vi "UI_VCH.vi"() -> ()   [LabVIEW 2016]
uses:
  <vilib>/Pansino Software/LabVIEW Architecture/Queue Management/PSARC_Queue Valid.vi
  <vilib>/Pansino Software/LabVIEW Architecture/Queue Management/PSARC_Queue Insert Element.vi
  <vilib>/Utility/error.llb/DialogType.ctl
  <vilib>/Pansino Software/LabVIEW Architecture/Queue Management/PSARC_Queue Remove Element.vi
  <vilib>/Pansino Software/LabVIEW Architecture/Queue Management/PSARC_Queue Destroy_Single.vi
  SubVIs/VCH/Private/Ctrls/PSVCH_VCH Status.ctl
  SubVIs/VCH/Private/Ctrls/PSVCH_All Channels.ctl
  SubVIs/VCH/Private/Ctrls/PSVCH_Status.ctl
  <vilib>/Pansino Software/LabVIEW Architecture/Queue Management/PSARC_Queue Create_Single.vi
  DAQ-Config/Controls/PSCHN_Channel Para.ctl
  DAQ-Config/Controls/PSCHN_Card Para.ctl
  <vilib>/Pansino Software/ToolkitLib/Popup Toolkit/Public/PSPOP_Popup Cluster.ctl
panel:
  in  "Caller":string
  in  "View":bool
  in  "Config":bool
  in  "Run":bool
  in  "Pause":bool
  in  "Stop":bool
  in  "Popups":T1 {"Time" format="%<%Y/%m/%d %I:%M:%S>T"; "Boolean" items=["False", "True"]; "Ring" items=["√", "×"]}
  in  "VCH":string(tree)
  out "Message":string caption="信息"
  # "Boolean Colors"
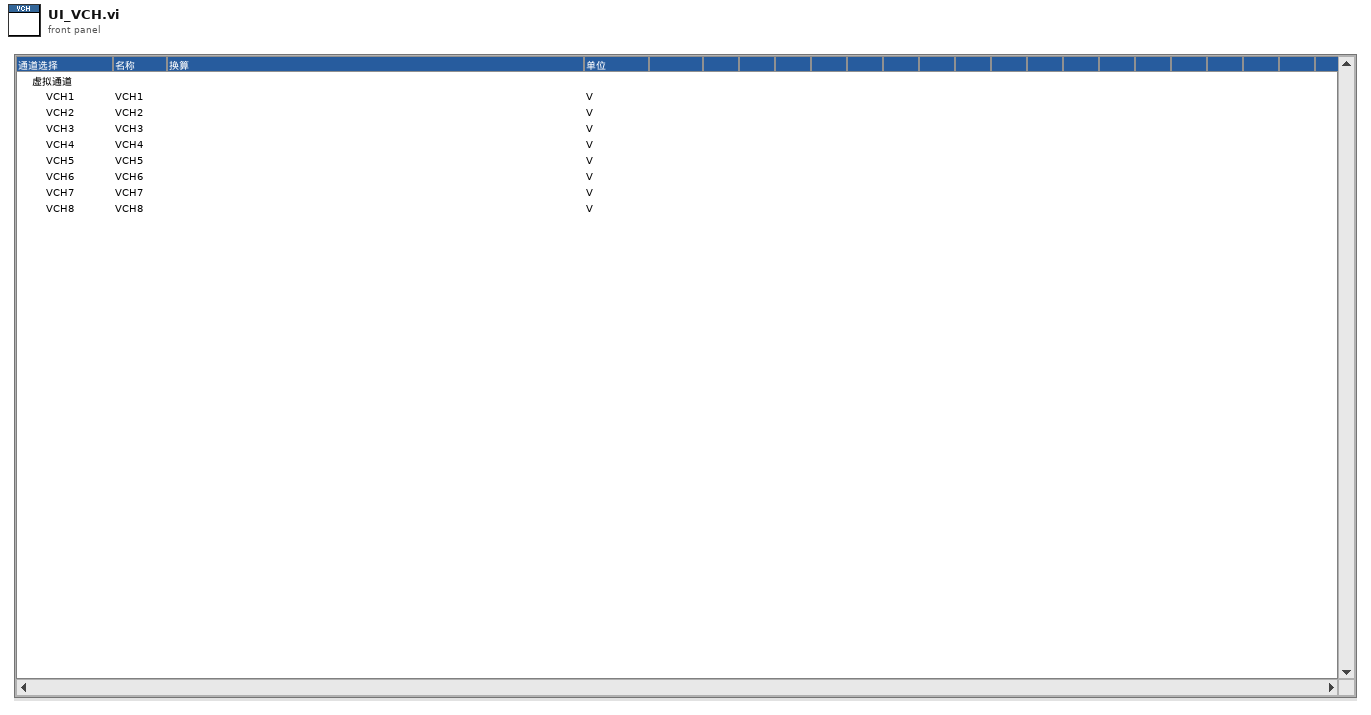
[diagram p1: front panel]
types:
  T1 = typedef "PSPOP_Popup Cluster.ctl" = cluster{"Unknown":bool, "Unknown 2":bool, "String":string, "Integer":i32, "Float":dbl, "Color":u32, "Boolean":u32, "Ring":u32, "Captioned String":cluster{"String":string, "OK":bool, "Cancel":bool}, "Captioned Integer":cluster{"First":i32, "OK":bool, "Cancel":bool}, "Boolean Colors":cluster{"False":cluster{"FG":u32, "BG":u32}, "True":cluster{"FG":u32, "BG":u32}, "T  to  F":cluster{"FG":u32, "BG":u32}, "F  to  T":cluster{"FG":u32, "BG":u32}, "OK":bool, "Cancel":bool}, "2-Int Cluster":cluster{"First":i32, "Second":i32, "OK":bool, "Cancel":bool}, "4-Int Cluster":cluster{"First":i32, "Second":i32, "Third":i32, "Fourth":i32, "OK":bool, "Cancel":bool}, "6-Dbl Cluster":cluster{"First":dbl, "Second":dbl, "Third":dbl, "Fourth":dbl, "Fourth 2":dbl, "Third 2":dbl, "OK":bool, "Cancel":bool}, "Path":path, "Combox":string, "Time":timestamp, "ShortCut":string}
  T2 = typedef "PSVCH_All Channels.ctl" = cluster{"Card Name":string, "Channels Tag":string[], "Channels Name":string[], "Unit":string[]}
  T3 = cluster{"Main Queue":string, "DAQ Queue":string, "ANA Queue":string, "CUI Queue":string, "Q-FocusList":string, "Q-Toolbar":string, "Q-Config":string}
  T4 = cluster{"Error":errorcluster, "Exit":bool, "Local VIRef":refnum<vi>, "Q_Local":cluster{"Name":string, "Order":string, "Data":variant}, "Q_High":cluster{"Name":string, "Order":string, "Data":variant}, "Q_Send":cluster{"Name[]":string[], "Order[]":string[], "Data[]":variant[]}, "Popup Index":i32, "Ref":cluster{"VCHList":refnum<vi>, "Message":refnum<vi>}, "Q_VCHEG":string, "DAQ2ANA":T2[], "PopUp Name":string, "Symbol Path":path}
  T5 = enum8{"Enabled", "Disabled", "Disabled and Grayed Out"}
  T6 = cluster{"Popup Value":variant, "Call Data":variant}
  T7 = typedef "PSVCH_VCH Status.ctl" = cluster{"Tag":string[], "Code[]":i32[], "Dispription[]":string[]}
  T8 = typedef "PSVCH_Status.ctl" = enum16{"Bad", "Stop", "Run", "Pause"}
  T9 = typedef "PSCHN_Card Para.ctl" = cluster{"Module Type":string, "Module Name":string, "ModuSN":string, "ModuIP":string, "Used?":bool, "Connected":bool, "Timing*":cluster{"Sample Rate":dbl}, "Channels":T10[]}
  T10 = typedef "PSCHN_Channel Para.ctl" = cluster{"CHTag*":string, "Used?*":bool, "CHName":string, "Unit":string, "斜率":dbl, "截距":dbl}
  T11 = cluster{"Queue":string, "DAQ Channels":string[]}[]
  T12 = typedef "DialogType.ctl" = u16
  T13 = typedef "PSVCH_VCH Info.ctl" = cluster{"Tag":string[], "Tag String":string[], "Name":string[], "Enable":bool[], "Formula":string[], "Unit":string[], "Save":bool[], "Time":i64[]}
  T14 = cluster{"Tag":string[], "Name":string[], "Type":variant[]}
  T15 = cluster{"VarList":cluster{"Tag":string[], "Name":string[], "Type":variant[]}, "VCH Out":T13}
  T16 = typedef "LVPoint32TypeDef.ctl" = cluster{"Horizontal":i32, "Vertical":i32}
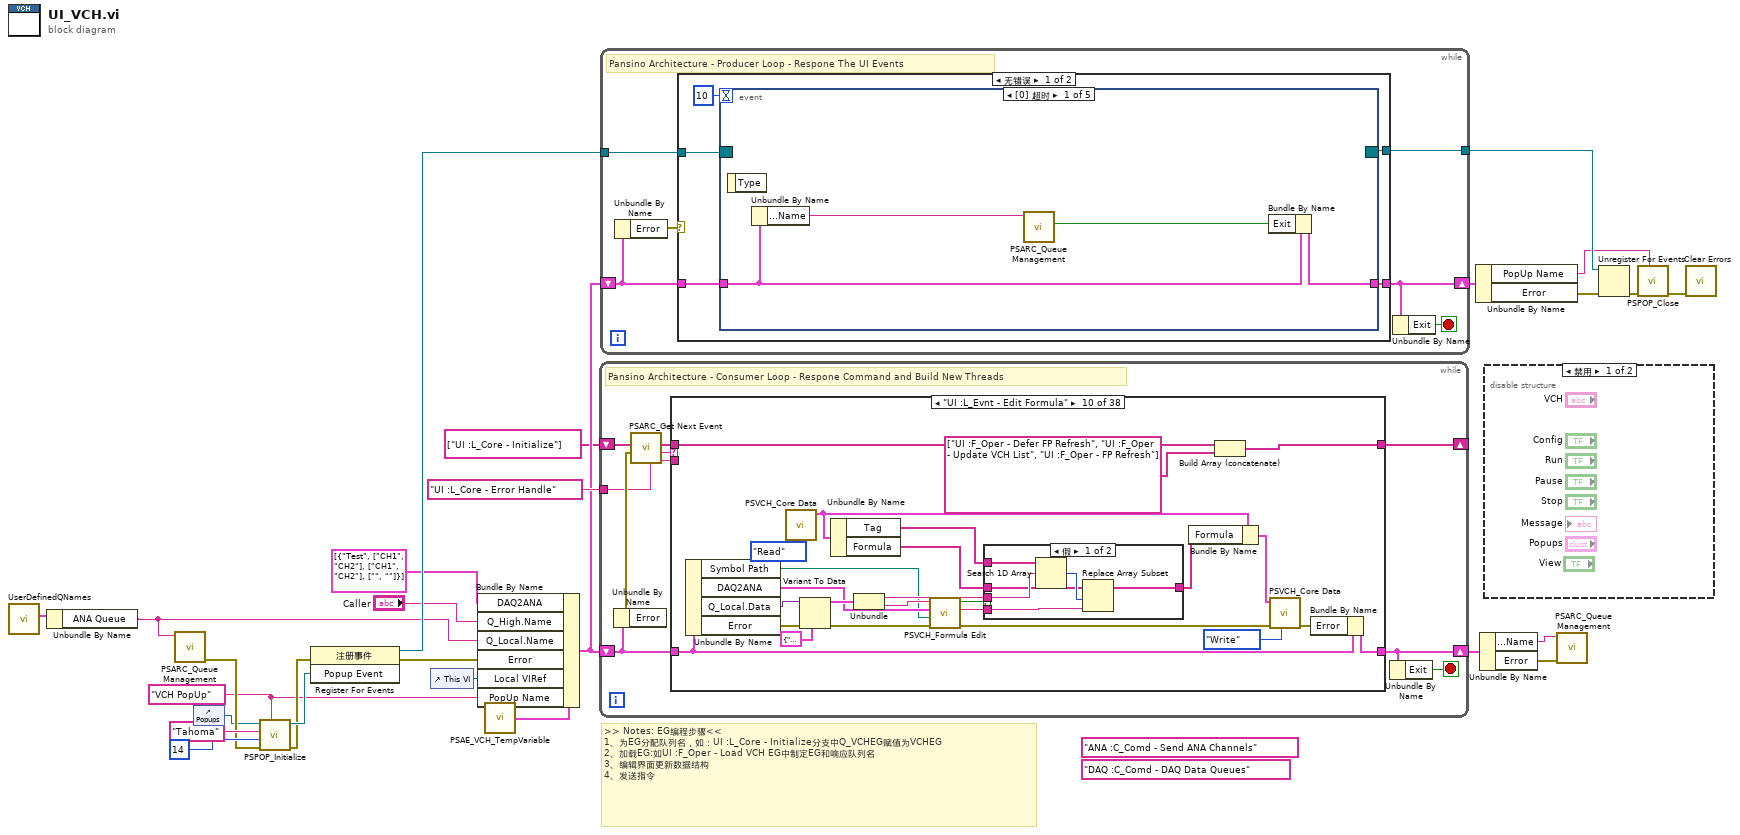
[diagram p0: block diagram]
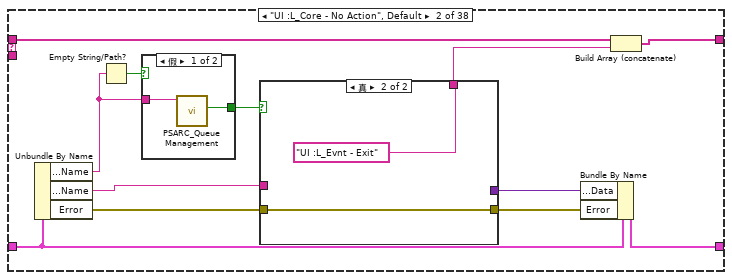
[diagram p4: hidden frame]
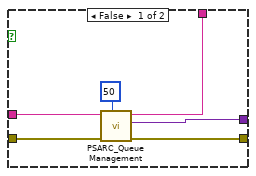
[diagram p6: hidden frame]
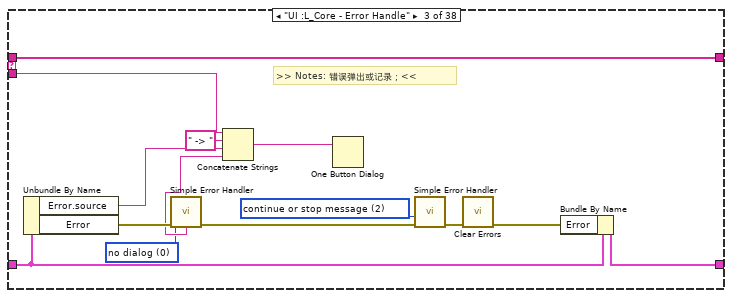
[diagram p7: hidden frame]
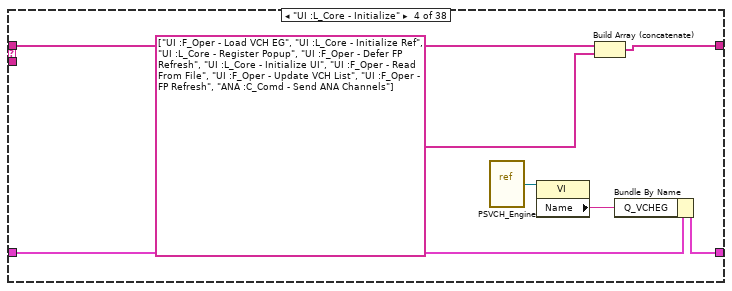
[diagram p8: hidden frame]
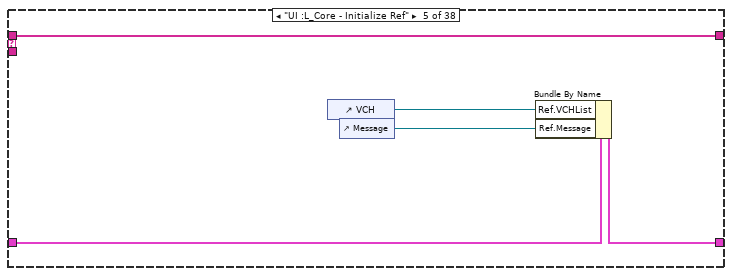
[diagram p9: hidden frame]
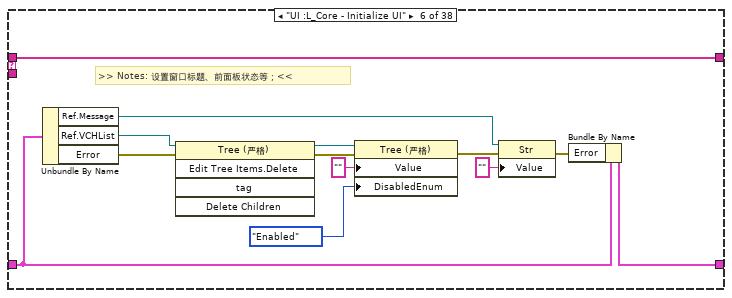
[diagram p10: hidden frame]
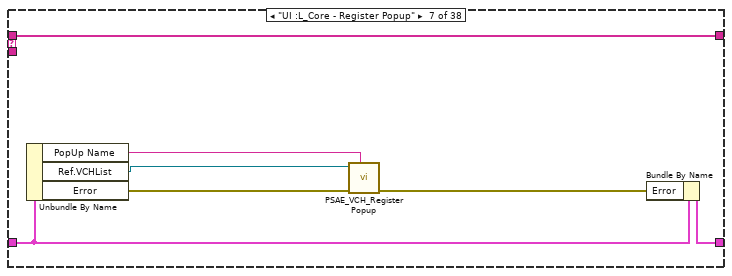
[diagram p11: hidden frame]
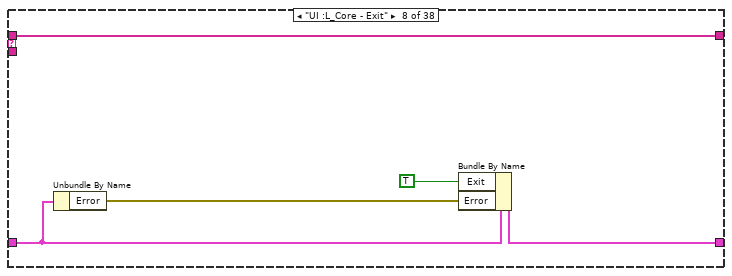
[diagram p12: hidden frame]
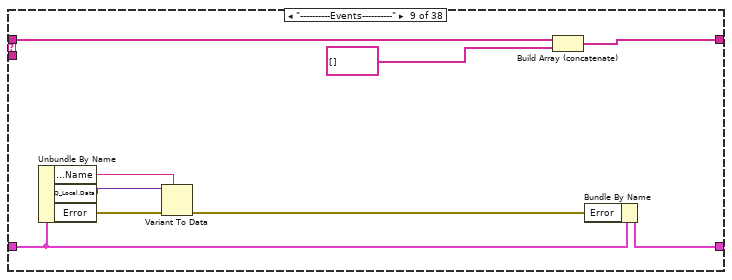
[diagram p13: hidden frame]
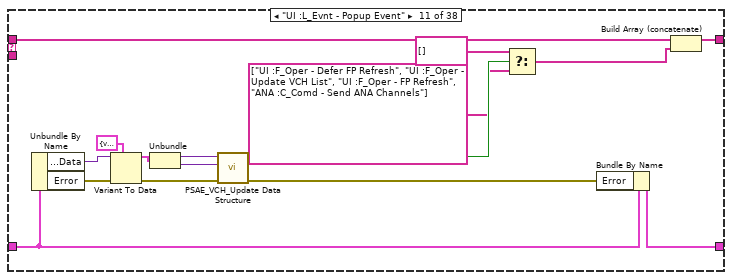
[diagram p15: hidden frame]
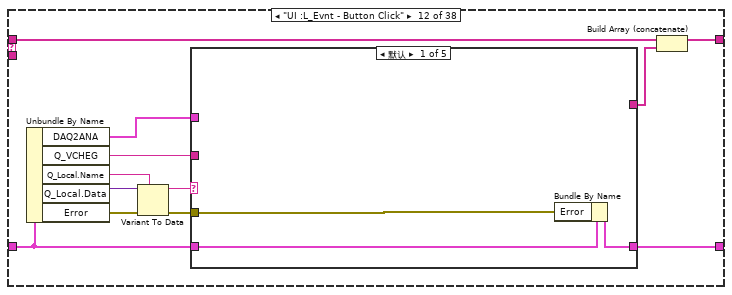
[diagram p16: hidden frame]
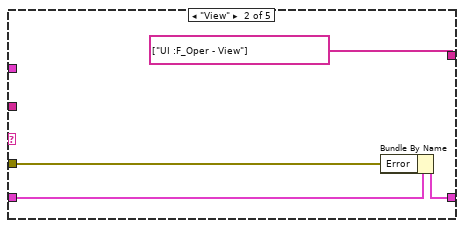
[diagram p17: hidden frame]
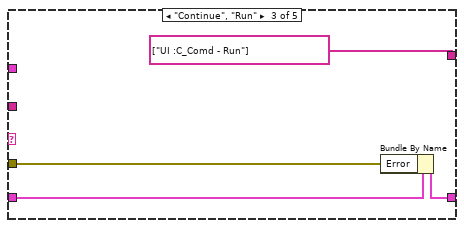
[diagram p18: hidden frame]
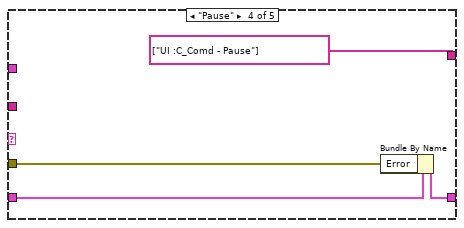
[diagram p19: hidden frame]
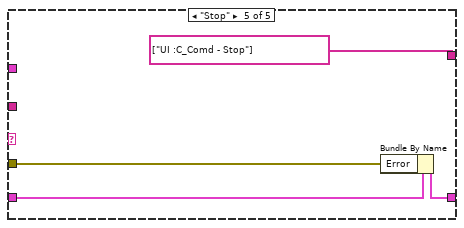
[diagram p20: hidden frame]
diagram:
  w4 = "VCH PopUp" ("Name")
  (unwired) "DAQ :C_Comd - DAQ Data Queues"
  (unwired) "ANA :C_Comd - Send ANA Channels"
  # ">> Notes: EG编程步骤<<\n1、为EG分配队列名，如：UI :L_Core - Initialize分支中Q_VCHEG赋值为VCHEG\n2、加载EG:如UI :F_Oper - Load VCH EG中制定EG和响应队列名\n3、编辑界面更新数据结构\n4、发送指令"
  n1 = call "UserDefinedQNames.vi"() -> ("All Queues"=w2:T3)  [unwired: 11 in]
  n2 = Unbundle By Name(w2) -> ("ANA Queue"=w1:string)
  n3 = call-poly <vilib>:"PSARC_Queue Management.vi"("Queue Name"=w1) -> ("error out"=w14:errorcluster)  [unwired: 9 in, 1 out]
  n4 = control-ref of="Popups"() -> (w13:refnum<vi>)
  n5 = call <vilib>:"PSPOP_Initialize.vi"("Name"=w4, "error in (no error)"=w14, "Font Size"=u32 14, "TontName"="Tahoma" ("Font Name"), "Popup Cluster Ref"=w13) -> ("error out"=w15:errorcluster, "Popup Event"=w19:refnum<user-event>)  [unwired: 5 in]
  n6 = register-events(error in=w15, w19) -> (reference out=w12:refnum<event-registration>, error out=w16:errorcluster)  [unwired: 1 in]
  n7 = control-ref of="This VI"() -> (w25:refnum<vi>)
  n8 = call "PSAE_VCH_TempVariable.vi"() -> ("TempVariable"=w20:T4)  [unwired: 5 in]
  n9 = Bundle By Name(cluster=w20, "DAQ2ANA"=T2[] [{"Card Name"="Test", "Channels Tag"=["CH1", "CH2"], "Channels Name"=["CH1", "CH2"], "Unit"=["", ""]}], "Q_High.Name"="Caller", "Q_Local.Name"=w1, "Error"=w16, "Local VIRef"=w25, "PopUp Name"=w4) -> (w26:T4)
  n10 = while {
    shift-right: [w31] -> w21
    shift-left: w26 -> [w33]
    shift-right: [w34] -> _
    shift-left: string[] ["UI :L_Core - Initialize"] -> [w37]
    tunnel: "UI :L_Core - Error Handle" ("Error Handle") -> [w29]
    stop <- w30 stop-if-true
    # "Pansino Architecture - Consumer Loop - Respone Command and Build New Threads"
    n11 = Unbundle By Name(w33) -> ("Error"=w32:errorcluster)
    n12 = call <vilib>:"PSARC_Get Next Event.vi"("Error Handle"=w29, "error in (no error)"=w32, "event queue in"=w37) -> ("prev event"=w28:string, "next event"=w36:string, "event queue out"=w35:string[])  [unwired: 3 in]
    n13 = case shown="\"UI :L_Evnt - Edit Formula\"" w36 {
      tunnel: w33 -> [w38 w48 w73 w81 w86 w99 w105 w109 w118 w143 w167 w173 w205 w265 w285 w295 w309 w321 w334 w346 w355 w365 w384 w403 w422 w431 w434 w447 w458 w465 w474 w491 w499 w506 w515 w532 w536 w546]
      tunnel: w35 -> [w39 w46 w75 w82 w87 w100 w107 w112 w121 w146 w169 w181 w213 w268 w288 w298 w317 w330 w343 w354 w358 w366 w367 w395 w423 w432 w435 w451 w462 w466 w475 w493 w500 w507 w516 w533 w537 w547]
      tunnel: [w39 w45 w75 w80 w87 w100 w107 w112 w120 w145 w168 w180 w212 w267 w287 w297 w316 w329 w342 w353 w357 w366 w367 w395 w423 w432 w435 w451 w462 w466 w475 w493 w500 w507 w516 w533 w537 w547] -> w34
      tunnel: [w38 w47 w74 w78 w85 w98 w103 w110 w117 w142 w166 w172 w204 w264 w289 w294 w311 w323 w336 w348 w355 w361 w383 w402 w418 w428 w433 w446 w457 w464 w468 w490 w498 w505 w514 w531 w535 w545] -> w31
      tunnel: w28 -> [_ _ w64 _ _ _ _ _ _ _ _ _ _ _ _ _ _ _ _ _ _ _ _ _ _ _ _ _ _ _ _ _ _ _ _ _ _ _]
      frame "----------Core Status----------" {
      }
      frame "UI :L_Core - No Action", Default {
        n14 = Unbundle By Name(w48) -> ("Q_High.Name"=w41:string, "Q_Local.Name"=w43:string, "Error"=w49:errorcluster)
        n15 = Empty String/Path?(string/path=w41) -> (empty?=w40:bool)
        n16 = case shown="假" w40 {
          tunnel: [w53 _] -> w42
          tunnel: w41 -> [w52 _]
          frame False {
            n17 = call-poly <vilib>:"PSARC_Queue Management.vi"("Queue Name(unamed)"=w52) -> ("Not Exist?"=w53:bool)  [unwired: 8 in, 2 out]
          }
          frame True {
          }
        }
        n18 = case shown="真" w42 {
          tunnel: [w59 w61] -> w51
          tunnel: [w58 _] -> w50
          tunnel: w49 -> [w57 w61]
          tunnel: [w56 "UI :L_Evnt - Exit" ("Event")] -> w44
          tunnel: w43 -> [w55 _]
          frame False {
            n19 = call-poly <vilib>:"PSARC_Queue Management.vi"("Time out(-1)_queue out"=50, "error in (no error)"=w57, "Queue Name(unamed)"=w55) -> ("error out"=w59:errorcluster, "Data"=w58:variant, "Event"=w56:string)  [unwired: 5 in, 1 out]
          }
          frame True {
          }
        }
        n20 = Bundle By Name(cluster=w48, "Q_Local.Data"=w50, "Error"=w51) -> (w47:T4)
        n21 = Build Array (concatenate)(w46, w44) -> (w45:string[])
      }
      frame "UI :L_Core - Error Handle" {
        w63 = T12 0 items=["no dialog", "OK message", "continue or stop message", "OK message + warnings", "continue/stop + warnings"] ("type of dialog (OK msg:1)")
        w70 = T12 2 items=["no dialog", "OK message", "continue or stop message", "OK message + warnings", "continue/stop + warnings"] ("type of dialog (OK msg:1)")
        # ">> Notes: 错误弹出或记录；<<"
        n22 = Unbundle By Name(w73) -> ("Error.source"=w65:string, "Error"=w68:errorcluster)
        n23 = call <vilib>:"Simple Error Handler.vi"("type of dialog (OK msg:1)"=w63, "error in (no error)"=w68) -> ("error out"=w67:errorcluster, "message"=w66:string)  [unwired: 3 in, 3 out]
        n24 = Concatenate Strings(w64, " -> " ("字符串"), w65, w66) -> (w62:string)
        n25 = One Button Dialog(message=w62) -> ()  [unwired: 1 in, 1 out]
        n26 = call <vilib>:"Simple Error Handler.vi"("type of dialog (OK msg:1)"=w70, "error in (no error)"=w67) -> ("error out"=w72:errorcluster)  [unwired: 3 in, 4 out]
        n27 = call <vilib>:"Clear Errors.vi"("error in (no error)"=w72) -> ("error out"=w71:errorcluster)  [unwired: 5 in, 1 out]
        n28 = Bundle By Name(cluster=w73, "Error"=w71) -> (w74:T4)
      }
      frame "UI :L_Core - Initialize" {
        n29 = vi-ref "PSVCH_Engine.vi"() -> (w77:refnum<vi>)
        n30 = property class="VI"(reference=w77) -> ("Name"=w76:string)  [unwired: 1 in, 2 out]
        n31 = Build Array (concatenate)(w82, string[] ["UI :F_Oper - Load VCH EG", "UI :L_Core - Initialize Ref", "UI :L_Core - Register Popup", "UI :F_Oper - Defer FP Refresh", "UI :L_Core - Initialize UI", "UI :F_Oper - Read From File", "UI :F_Oper - Update VCH List", "UI :F_Oper - FP Refresh", "ANA :C_Comd - Send ANA Channels"] ("数组")) -> (w80:string[])
        n32 = Bundle By Name(cluster=w81, "Q_VCHEG"=w76) -> (w78:T4)
      }
      frame "UI :L_Core - Initialize Ref" {
        n33 = control-ref of="VCH"() -> (w84:refnum<vi>)
        n34 = control-ref of="Message"() -> (w83:refnum<vi>)
        n35 = Bundle By Name(cluster=w86, "Ref.VCHList"=w84, "Ref.Message"=w83) -> (w85:T4)
      }
      frame "UI :L_Core - Initialize UI" {
        # ">> Notes: 设置窗口标题、前面板状态等；<<"
        n36 = Unbundle By Name(w99) -> ("Ref.Message"=w97:refnum<vi>, "Ref.VCHList"=w91:refnum<vi>, "Error"=w90:errorcluster)
        n37 = invoke class="Tree (严格)" method="Edit Tree Items.Delete"(reference=w91, error in=w90) -> (reference out=w93:refnum<vi>, error out=w92:errorcluster)  [unwired: 3 in, 3 out]
        n38 = property class="Tree (严格)"(reference=w93, error in=w92, "Value"="" ("值"), "DisabledEnum"=T5."Enabled" ("Disabled")) -> (error out=w94:errorcluster)  [unwired: 1 out]
        n39 = property class="Str"(reference=w97, error in=w94, "Value"="" ("值")) -> (error out=w95:errorcluster)  [unwired: 1 out]
        n40 = Bundle By Name(cluster=w99, "Error"=w95) -> (w98:T4)
      }
      frame "UI :L_Core - Register Popup" {
        n41 = Unbundle By Name(w105) -> ("PopUp Name"=w101:string, "Ref.VCHList"=w104:refnum<vi>, "Error"=w106:errorcluster)
        n42 = call "PSAE_VCH_Register Popup.vi"("PopUp Name"=w101, "Error In (no error)"=w106, "Tree Ref"=w104) -> ("Error Out"=w102:errorcluster)  [unwired: 8 in]
        n43 = Bundle By Name(cluster=w105, "Error"=w102) -> (w103:T4)
      }
      frame "UI :L_Core - Exit" {
        n44 = Unbundle By Name(w109) -> ("Error"=w111:errorcluster)
        n45 = Bundle By Name(cluster=w109, "Exit"=TRUE, "Error"=w111) -> (w110:T4)
      }
      frame "----------Events----------" {
        n46 = Unbundle By Name(w118) -> ("Q_Local.Name"=w113:string, "Q_Local.Data"=w114:variant, "Error"=w116:errorcluster)
        n47 = Variant To Data(error in=w116, type=w113, Variant=w114) -> (error out=w115:errorcluster)  [unwired: 1 out]
        n48 = Build Array (concatenate)(w121, string[] [] ("数组")) -> (w120:string[])
        n49 = Bundle By Name(cluster=w118, "Error"=w115) -> (w117:T4)
      }
      frame "UI :L_Evnt - Edit Formula" {
        n50 = Unbundle By Name(w143) -> ("Symbol Path"=w124:path, "DAQ2ANA"=w132:T2[], "Q_Local.Data"=w140:variant, "Error"=w141:errorcluster)
        n51 = call "PSVCH_Core Data.vi"("Oper"=enum16{"Init", "Read", "Write"}."Read") -> ("VCH Out"=w129:T13)  [unwired: 9 in, 1 out]
        n52 = Variant To Data(error in=w141, type=cluster{"Tag":string, "Cell String":string} {"Tag"="", "Cell String"=""} ("输出簇"), Variant=w140) -> (data=w137:cluster{"Tag":string, "Cell String":string}, error out=w138:errorcluster)
        n53 = Unbundle By Name(w129) -> ("Tag"=w131:string[], "Formula"=w130:string[])
        n54 = Unbundle(w137) -> ("Tag"=w133:string, "Cell String"=w136:string)
        n55 = call "PSVCH_Formula Edit.vi"("Error In (no error)"=w138, "Symbol Path"=w124, "DAQ2ANA"=w132, "Formula In"=w136) -> ("Error Out"=w125:errorcluster, "Formula"=w134:string, "Cancel?"=w135:bool)  [unwired: 5 in]
        n56 = case shown="假" w135 {
          tunnel: w134 -> [w148 _]
          tunnel: w131 -> [w152 _]
          tunnel: w130 -> [w149 w153]
          tunnel: [w147 w153] -> w128
          tunnel: w133 -> [w151 _]
          frame False {
            n57 = Search 1D Array(1D array=w152, element=w151) -> (index of element=w150:i32)  [unwired: 1 in]
            n58 = Replace Array Subset(array=w149, new element=w148, index=w150) -> (w147:string[])
          }
          frame True {
          }
        }
        n59 = Bundle By Name(cluster=w129, "Formula"=w128) -> (w127:T13)
        n60 = Build Array (concatenate)(w146, string[] ["UI :F_Oper - Defer FP Refresh", "UI :F_Oper - Update VCH List", "UI :F_Oper - FP Refresh"] ("数组")) -> (w145:string[])
        n61 = call "PSVCH_Core Data.vi"("Oper"=enum16{"Init", "Read", "Write"}."Write", "Error In (no error)"=w125, "VCH In"=w127) -> ("Error Out"=w126:errorcluster)  [unwired: 7 in, 1 out]
        n62 = Bundle By Name(cluster=w143, "Error"=w126) -> (w142:T4)
      }
      frame "UI :L_Evnt - Popup Event" {
        n63 = Unbundle By Name(w167) -> ("Q_Local.Data"=w164:variant, "Error"=w165:errorcluster)
        n64 = Variant To Data(error in=w165, type=T6 {"Popup Value"=variant, "Call Data"=variant} ("输出簇"), Variant=w164) -> (data=w162:T6, error out=w159:errorcluster)
        n65 = Unbundle(w162) -> ("Popup Value"=w161:variant, "Call Data"=w160:variant)
        n66 = call "PSAE_VCH_Update Data Structure.vi"("Error In (no error)"=w159, "Call Data"=w160, "Popup Value"=w161) -> ("Error Out"=w158:errorcluster, "Giveup？"=w157:bool)  [unwired: 7 in]
        n67 = Select(t=string[] [], s=w157, f=string[] ["UI :F_Oper - Defer FP Refresh", "UI :F_Oper - Update VCH List", "UI :F_Oper - FP Refresh", "ANA :C_Comd - Send ANA Channels"] ("数组")) -> (s? t:f=w155:string[])
        n68 = Bundle By Name(cluster=w167, "Error"=w158) -> (w166:T4)
        n69 = Build Array (concatenate)(w169, w155) -> (w168:string[])
      }
      frame "UI :L_Evnt - Button Click" {
        n70 = Unbundle By Name(w173) -> ("DAQ2ANA"=w170:T2[], "Q_VCHEG"=w174:string, "Q_Local.Name"=w176:string, "Q_Local.Data"=w177:variant, "Error"=w178:errorcluster)
        n71 = Variant To Data(error in=w178, type=w176, Variant=w177) -> (data=w175:string, error out=w171:errorcluster)
        n72 = case shown="默认" w175 {
          tunnel: [_ string[] ["UI :F_Oper - View"] ("数组") string[] ["UI :C_Comd - Run"] ("数组") string[] ["UI :C_Comd - Pause"] ("数组") string[] ["UI :C_Comd - Stop"] ("数组")] -> w179
          tunnel: w174 -> [_ _ _ _ _]
          tunnel: w173 -> [w184 w187 w191 w195 w199]
          tunnel: [w183 w186 w190 w194 w198] -> w172
          tunnel: w171 -> [w182 w185 w189 w193 w197]
          tunnel: w170 -> [_ _ _ _ _]
          frame Default {
            n73 = Bundle By Name(cluster=w184, "Error"=w182) -> (w183:T4)
          }
          frame "View" {
            n74 = Bundle By Name(cluster=w187, "Error"=w185) -> (w186:T4)
          }
          frame "Continue", "Run" {
            n75 = Bundle By Name(cluster=w191, "Error"=w189) -> (w190:T4)
          }
          frame "Pause" {
            n76 = Bundle By Name(cluster=w195, "Error"=w193) -> (w194:T4)
          }
          frame "Stop" {
            n77 = Bundle By Name(cluster=w199, "Error"=w197) -> (w198:T4)
          }
        }
        n78 = Build Array (concatenate)(w181, w179) -> (w180:string[])
      }
      frame "UI :L_Evnt - Button Click*" {
        n79 = Unbundle By Name(w205) -> ("DAQ2ANA"=w202:T2[], "Q_VCHEG"=w206:string, "Q_Local.Name"=w208:string, "Q_Local.Data"=w209:variant, "Error"=w210:errorcluster)
        n80 = call "PSVCH_Core Data.vi"() -> ("VCH Out"=w201:T13)  [unwired: 10 in, 1 out]
        n81 = Variant To Data(error in=w210, type=w208, Variant=w209) -> (data=w207:string, error out=w203:errorcluster)
        n82 = case shown="\"View\"" w207 {
          selector: w207 -> [_ w226 w242 _]
          tunnel: [_ string[] ["UI :F_Oper - Send To Threads"] ("数组") string[] ["UI :F_Oper - Send To Threads"] ("数组") string[] ["UI :F_Oper - View"] ("数组")] -> w211
          tunnel: w206 -> [_ w225 w241 _]
          tunnel: w205 -> [w216 w222 w239 w247]
          tunnel: [w215 w221 w238 w246] -> w204
          tunnel: w203 -> [w214 w217 w234 w245]
          tunnel: w201 -> [_ _ w233 _]
          tunnel: w202 -> [_ _ w230 _]
          frame Default {
            n83 = Bundle By Name(cluster=w216, "Error"=w214) -> (w215:T4)
          }
          frame "Continue", "Pause", "Run", "Stop" {
            n84 = Concatenate Strings("UI :C_Comd - ", w226) -> (w224:string)
            n85 = Build Array(w225) -> (w220:string[])
            n86 = Build Array(w224) -> (w219:string[])
            n87 = Build Array(variant ("Variant")) -> (w218:variant[])
            n88 = Bundle By Name(cluster=w222, "Q_Send.Name[]"=w220, "Q_Send.Order[]"=w219, "Q_Send.Data[]"=w218, "Error"=w217) -> (w221:T4)
          }
          frame "Config" {
            n89 = call "PSVCH_Convert Data.vi"("DAQ2ANA"=w230) -> ("VarList"=w229:T14)  [unwired: 10 in]
            n90 = Bundle("VarList"=w229, "VCH Out"=w233) -> (w231:T15)  [unwired: 1 in]
            n91 = Concatenate Strings("UI :C_Comd - ", w242) -> (w240:string)
            n92 = To Variant(anything=w231) -> (Variant=w232:variant)
            n93 = Build Array(w241) -> (w237:string[])
            n94 = Build Array(w240) -> (w236:string[])
            n95 = Build Array(w232) -> (w235:variant[])
            n96 = Bundle By Name(cluster=w239, "Q_Send.Name[]"=w237, "Q_Send.Order[]"=w236, "Q_Send.Data[]"=w235, "Error"=w234) -> (w238:T4)
          }
          frame "View" {
            n97 = Bundle By Name(cluster=w247, "Error"=w245) -> (w246:T4)
          }
        }
        n98 = Build Array (concatenate)(w213, w211) -> (w212:string[])
      }
      frame "UI :L_Evnt - Click VCH Symbol" {
        n99 = Unbundle By Name(w265) -> ("Q_Local.Name"=w261:string, "Q_Local.Data"=w262:variant, "Error"=w263:errorcluster)
        n100 = Variant To Data(error in=w263, type=w261, Variant=w262) -> (data=w260:string, error out=w256:errorcluster)
        n101 = call "PSVCH_Core Data.vi"("Oper"=enum16{"Init", "Read", "Write"}."Read", "Error In (no error)"=w256) -> ("Error Out"=w255:errorcluster, "VCH Out"=w253:T13)  [unwired: 8 in]
        n102 = Unbundle By Name(w253) -> ("Enable"=w258:bool[], "Tag"=w257:string[])
        n103 = Search 1D Array(1D array=w257, element=w260) -> (index of element=w259:i32)  [unwired: 1 in]
        n104 = case shown="默认" w259 {
          selector: w259 -> [_ w274]
          tunnel: w258 -> [w273 w277]
          tunnel: [w271 w275] -> w254
          frame -1 {
            n105 = And Array Elements(Boolean array=w273) -> (logical AND=w270:bool)
            n106 = Array Size(array=w273) -> (size(s)=w272:i32)
            n107 = Not(x=w270) -> (.not. x?=w269:bool)
            n108 = Initialize Array(w269, w272) -> (w271:bool[])
          }
          frame Default {
            n109 = Index Array(array=w277, index=w274) -> (element=w278:bool)
            n110 = Not(x=w278) -> (.not. x?=w276:bool)
            n111 = Replace Array Subset(array=w277, new element=w276, index=w274) -> (w275:bool[])
          }
        }
        n112 = Bundle By Name(cluster=w253, "Enable"=w254) -> (w252:T13)
        n113 = call "PSVCH_Core Data.vi"("Oper"=enum16{"Init", "Read", "Write"}."Write", "Error In (no error)"=w255, "VCH In"=w252) -> ("Error Out"=w251:errorcluster)  [unwired: 7 in, 1 out]
        n114 = Build Array (concatenate)(w268, string[] ["UI :F_Oper - Defer FP Refresh", "UI :F_Oper - Update VCH List", "UI :F_Oper - FP Refresh", "ANA :C_Comd - Send ANA Channels"] ("数组")) -> (w267:string[])
        n115 = Bundle By Name(cluster=w265, "Error"=w251) -> (w264:T4)
      }
      frame "UI :L_Evnt - Exit" {
        n116 = Unbundle By Name(w285) -> ("Q_VCHEG"=w284:string)
        n117 = Build Array(w284) -> (w283:string[])
        n118 = Build Array("UI :C_Comd - Exit" ("Q_VCHEG")) -> (w282:string[])
        n119 = Build Array(variant ("Variant")) -> (w280:variant[])
        n120 = Bundle By Name(cluster=w285, "Q_Send.Name[]"=w283, "Q_Send.Order[]"=w282, "Q_Send.Data[]"=w280) -> (w289:T4)
        n121 = Build Array (concatenate)(w288, string[] ["UI :F_Oper - Send To Threads", "UI :L_Core - Exit"] ("数组")) -> (w287:string[])
      }
      frame "----------Communications----------" {
        n122 = Unbundle By Name(w295) -> ("Q_Local.Name"=w290:string, "Q_Local.Data"=w291:variant, "Error"=w293:errorcluster)
        n123 = Variant To Data(error in=w293, type=w290, Variant=w291) -> (error out=w292:errorcluster)  [unwired: 1 out]
        n124 = Build Array (concatenate)(w298, string[] [] ("数组")) -> (w297:string[])
        n125 = Bundle By Name(cluster=w295, "Error"=w292) -> (w294:T4)
      }
      frame "UI :C_Comd - Run" {
        n126 = Unbundle By Name(w309) -> ("Ref.VCHList"=w300:refnum<vi>, "Q_VCHEG"=w310:string, "DAQ2ANA"=w307:T2[], "Error"=w304:errorcluster)
        n127 = call "PSVCH_Convert Data.vi"("DAQ2ANA"=w307) -> ("VarList"=w306:T14)  [unwired: 10 in]
        n128 = call "PSVCH_Core Data.vi"("Error In (no error)"=w304) -> ("Error Out"=w301:errorcluster, "VCH Out"=w305:T13)  [unwired: 9 in]
        n129 = Bundle("VarList"=w306, "VCH Out"=w305) -> (w303:T15)  [unwired: 1 in]
        n130 = property class="Tree (严格)"(reference=w300, "DisabledEnum"=T5."Disabled and Grayed Out" ("Disabled")) -> ()  [unwired: 1 in, 2 out]
        n131 = To Variant(anything=w303) -> (Variant=w302:variant)
        n132 = Build Array(w310) -> (w314:string[])
        n133 = Build Array("UI :C_Comd - Start") -> (w313:string[])
        n134 = Build Array(w302) -> (w312:variant[])
        n135 = Build Array (concatenate)(w317, string[] ["UI :F_Oper - Send To Threads"] ("数组")) -> (w316:string[])
        n136 = Bundle By Name(cluster=w309, "Q_Send.Name[]"=w314, "Q_Send.Order[]"=w313, "Q_Send.Data[]"=w312, "Error"=w301) -> (w311:T4)
      }
      frame "UI :C_Comd - Pause" {
        n137 = Unbundle By Name(w321) -> ("Ref.VCHList"=w318:refnum<vi>, "Q_VCHEG"=w322:string)
        n138 = property class="Tree (严格)"(reference=w318, "DisabledEnum"=T5."Disabled and Grayed Out" ("Disabled")) -> ()  [unwired: 1 in, 2 out]
        n139 = Build Array(w322) -> (w326:string[])
        n140 = Build Array("UI :C_Comd - Pause") -> (w325:string[])
        n141 = Build Array(variant ("Variant")) -> (w324:variant[])
        n142 = Build Array (concatenate)(w330, string[] ["UI :F_Oper - Send To Threads"] ("数组")) -> (w329:string[])
        n143 = Bundle By Name(cluster=w321, "Q_Send.Name[]"=w326, "Q_Send.Order[]"=w325, "Q_Send.Data[]"=w324) -> (w323:T4)
      }
      frame "UI :C_Comd - Stop" {
        n144 = Unbundle By Name(w334) -> ("Ref.VCHList"=w331:refnum<vi>, "Q_VCHEG"=w335:string)
        n145 = property class="Tree (严格)"(reference=w331, "DisabledEnum"=T5."Enabled" ("Disabled")) -> ()  [unwired: 1 in, 2 out]
        n146 = Build Array(w335) -> (w339:string[])
        n147 = Build Array("UI :C_Comd - Stop") -> (w338:string[])
        n148 = Build Array(variant ("Variant")) -> (w337:variant[])
        n149 = Build Array (concatenate)(w343, string[] ["UI :F_Oper - Send To Threads"] ("数组")) -> (w342:string[])
        n150 = Bundle By Name(cluster=w334, "Q_Send.Name[]"=w339, "Q_Send.Order[]"=w338, "Q_Send.Data[]"=w337) -> (w336:T4)
      }
      frame "UI :C_Comd - Save" {
        n151 = Unbundle By Name(w346) -> ("Q_VCHEG"=w347:string, "Q_Local.Data"=w344:variant)
        n152 = Build Array(w347) -> (w351:string[])
        n153 = Build Array("UI :C_Comd - Save") -> (w350:string[])
        n154 = Build Array(w344) -> (w349:variant[])
        n155 = Build Array (concatenate)(w354, string[] ["UI :F_Oper - Send To Threads"] ("数组")) -> (w353:string[])
        n156 = Bundle By Name(cluster=w346, "Q_Send.Name[]"=w351, "Q_Send.Order[]"=w350, "Q_Send.Data[]"=w349) -> (w348:T4)
      }
      frame "UI :C_Comd - Update Data" {
        n157 = Build Array (concatenate)(w358, string[] ["UI :F_Oper - Update VCH List"] ("数组")) -> (w357:string[])
      }
      frame "UI :C_Comd - Symbol Path" {
        # "谁给这个线程发的？？"
        n158 = Unbundle By Name(w365) -> ("Symbol Path"=w362:path, "Q_Local.Data"=w363:variant, "Error"=w364:errorcluster)
        n159 = Variant To Data(error in=w364, type=w362, Variant=w363) -> (data=w359:path, error out=w360:errorcluster)
        n160 = Bundle By Name(cluster=w365, "Symbol Path"=w359, "Error"=w360) -> (w361:T4)
      }
      frame "VCHEG :C_Resp - Config*" {
        # ">> Notes: 返回状态、错误代码及描述，添加处理返回状态的代码，本例直接显示在字符串控件中；<<"
        n161 = Unbundle By Name(w384) -> ("Ref.Message"=w368:refnum<vi>, "Q_Local.Data"=w381:variant, "Error"=w382:errorcluster)
        n162 = Variant To Data(error in=w382, type=T7 {"Tag"=[], "Code[]"=[], "Dispription[]"=[]} ("输出簇"), Variant=w381) -> (data=w371:T7, error out=w370:errorcluster)
        n163 = Unbundle(w371) -> ("Tag"=w375:string[], "Code[]"=w374:i32[], "Dispription[]"=w373:string[])
        n164 = for {
          tunnel: [w389] -> w376 mode=indexing
          tunnel: w375 -> [w388] mode=indexing
          tunnel: w374 -> [w387] mode=indexing
          tunnel: w373 -> [w386] mode=indexing
          tunnel: ">>%s:%d-%s" ("初始字符串") -> [w385]
          n165 = Format Into String(format string=w385, w388, w387, w386) -> (resulting string=w389:string)  [unwired: 2 in, 1 out]
        }
        n166 = Array To Spreadsheet String(delimiter (Tab)="\n", array=w376, 3:"%s" ("格式字符串")) -> (spreadsheet string=w369:string)
        n167 = property class="Str"(reference=w368, error in=w370, "Value"=w369) -> (error out=w379:errorcluster)  [unwired: 1 out]
        n168 = Bundle By Name(cluster=w384, "Error"=w379) -> (w383:T4)
      }
      frame "VCHEG :C_Resp - Config" {
        # ">> Notes: 返回状态、错误代码及描述，添加处理返回状态的代码，本例直接显示在字符串控件中；<<"
        n169 = Unbundle By Name(w403) -> ("Q_Local.Data"=w400:variant, "Error"=w401:errorcluster)
        n170 = Variant To Data(error in=w401, type=T7 {"Tag"=[], "Code[]"=[], "Dispription[]"=[]} ("输出簇"), Variant=w400) -> (data=w396:T7, error out=w390:errorcluster)
        n171 = Unbundle(w396) -> ("Tag"=w398:string[], "Code[]"=w394:i32[], "Dispription[]"=w397:string[])
        n172 = Equal?(x=0, y=w394) -> (x = y?=w392:bool[])
        n173 = And Array Elements(Boolean array=w392) -> (logical AND=w391:bool)
        n174 = case shown="假" w391 {
          tunnel: w398 -> [w408 _]
          tunnel: w397 -> [w407 _]
          tunnel: w394 -> [w405 _]
          frame False {
            n175 = for {
              tunnel: [w416] -> w409 mode=indexing
              tunnel: w408 -> [w415] mode=indexing
              tunnel: w405 -> [w414] mode=indexing
              tunnel: w407 -> [w413] mode=indexing
              tunnel: ">>%s:%d-%s" ("初始字符串") -> [w412]
              n176 = Format Into String(format string=w412, w415, w414, w413) -> (resulting string=w416:string)  [unwired: 2 in, 1 out]
            }
            n177 = Array To Spreadsheet String(delimiter (Tab)="\n", array=w409, 3:"%s" ("格式字符串")) -> (spreadsheet string=w404:string)
            n178 = One Button Dialog(message=w404) -> ()  [unwired: 1 in, 1 out]
          }
          frame True {
          }
        }
        n179 = Bundle By Name(cluster=w403, "Error"=w390) -> (w402:T4)
      }
      frame "VCHEG :C_Resp - Status" {
        n180 = Unbundle By Name(w422) -> ("Q_Local.Data"=w420:variant, "Error"=w421:errorcluster)
        n181 = Variant To Data(error in=w421, type=PSVCH_Status."Bad" ("Execute.Run Status"), Variant=w420) -> (error out=w417:errorcluster)  [unwired: 1 out]
        n182 = Bundle By Name(cluster=w422, "Error"=w417) -> (w418:T4)
      }
      frame "VCHEG :C_Resp - Error" {
        n183 = Unbundle By Name(w431) -> ("Error"=w427:errorcluster, "Q_Local.Data"=w429:variant, "Error"=w430:errorcluster)
        n184 = Variant To Data(error in=w430, type=w427, Variant=w429) -> (data=w425:errorcluster, error out=w426:errorcluster)
        n185 = Merge Errors(w425, w426) -> (w424:errorcluster)
        n186 = Bundle By Name(cluster=w431, "Error"=w424) -> (w428:T4)
      }
      frame "COM : DAQ_CFG Updata" {
        n187 = disable-structure shown="默认" {
          disable-tunnel: w434 -> [w443 w444]
          disable-tunnel: [w442 w444] -> w433
          frame condition #0 (active) {
            # "cards"
            n188 = Unbundle By Name(w443) -> ("Q_Local.Data"=w441:variant, "Error"=w440:errorcluster)
            n189 = Variant To Data(error in=w440, type=T9[] [] ("Cards"), Variant=w441) -> (data=w437:T9[], error out=w439:errorcluster)
            n190 = call "PSCHN_Convert Cards To CHInfo.vi"("Cards"=w437) -> ("VCH"=w436:T2[])  [unwired: 10 in]
            n191 = Bundle By Name(cluster=w443, "DAQ2ANA"=w436, "Error"=w439) -> (w442:T4)
          }
          frame condition #1 {
          }
        }
      }
      frame "DAQ :C_Comd - DAQ Data Queues" {
        n192 = Unbundle By Name(w447) -> ("Q_Local.Data"=w450:variant, "Error"=w449:errorcluster)
        n193 = Variant To Data(error in=w449, type=T11 [] ("DAQ DATA"), Variant=w450) -> (error out=w448:errorcluster)  [unwired: 1 out]
        n194 = Bundle By Name(cluster=w447, "Error"=w448) -> (w446:T4)
      }
      frame "ANA :C_Comd - Send ANA Channels" {
        # ">> Notes: 此处发送通道信息到显示界面模块；初始化和变更时发送。<<"
        n195 = Unbundle By Name(w458) -> ("Error"=w459:errorcluster)
        n196 = call "PSAE_VCH_VCH List.vi"("Error In (no error)"=w459) -> ("Error Out"=w461:errorcluster, "VCHList"=w460:T2)  [unwired: 9 in]
        n197 = call "UserDefinedQNames.vi"() -> ("All Queues"=w455:T3)  [unwired: 11 in]
        n198 = To Variant(anything=w460) -> (Variant=w452:variant)
        n199 = Unbundle By Name(w455) -> ("Main Queue"=w456:string)
        n200 = call <vilib>:"PSARC_Insert Single Messenges.vi"("error in (no error)"=w461, "Data"=w452, "Order"="COM : VCH_CFG Updata", "Queue Name"=w456) -> ("error out"=w454:errorcluster)  [unwired: 7 in]
        n201 = Bundle By Name(cluster=w458, "Error"=w454) -> (w457:T4)
      }
      frame "----------Operations----------" {
        n202 = Unbundle By Name(w465) -> ("Error"=w463:errorcluster)
        n203 = Bundle By Name(cluster=w465, "Error"=w463) -> (w464:T4)
      }
      frame "UI :F_Oper - Send To Threads" {
        n204 = Unbundle By Name(w474) -> ("Q_Send.Name[]"=w473:string[], "Q_Send.Order[]"=w472:string[], "Q_Send.Data[]"=w471:variant[], "Error"=w470:errorcluster)
        n205 = for {
          tunnel: w473 -> [w476] mode=indexing
          tunnel: w472 -> [w480] mode=indexing
          tunnel: w471 -> [w479] mode=indexing
          tunnel: w470 -> [w478]
          tunnel: [w477] -> w469 mode=indexing
          n206 = call-poly <vilib>:"PSARC_Queue Management.vi"("Queue Name(unamed)"=w476) -> ("Not Exist?"=w481:bool)  [unwired: 8 in, 2 out]
          n207 = case shown="假" w481 {
            tunnel: w476 -> [w486 _]
            tunnel: w480 -> [w485 _]
            tunnel: w479 -> [w484 _]
            tunnel: w478 -> [w483 w487]
            tunnel: [w482 w487] -> w477
            frame False {
              n208 = call-poly <vilib>:"PSARC_Queue Management.vi"("error in (no error)"=w483, "Data"=w484, "Event"=w485, "Queue Name(unamed)"=w486) -> ("error out"=w482:errorcluster)  [unwired: 6 in, 1 out]
            }
            frame True {
            }
          }
        }
        n209 = Merge Errors(w469) -> (w467:errorcluster)
        n210 = Bundle By Name(cluster=w474, "Error"=w467) -> (w468:T4)
      }
      frame "UI :F_Oper - Read From File" {
        # ">> Notes: 从配置文件中读取配置信息，此处暂时给常量；<<"
        n211 = Unbundle By Name(w491) -> ("Error"=w492:errorcluster)
        n212 = call "PSVCH_Core Data.vi"("Oper"=enum16{"Init", "Read", "Write"}."Init", "Error In (no error)"=w492) -> ("Error Out"=w489:errorcluster)  [unwired: 8 in, 1 out]
        n213 = Bundle By Name(cluster=w491, "Error"=w489) -> (w490:T4)
      }
      frame "UI :F_Oper - Defer FP Refresh" {
        # ">> Notes: 延迟前面板刷新；<<"
        n214 = Unbundle By Name(w499) -> ("Local VIRef"=w495:refnum<vi>, "Error"=w497:errorcluster)
        n215 = call <vilib>:"PSGEN_Front Panel Delay.vi"("error in (no error)"=w497, "Delay?"=TRUE ("Defer"), "VI"=w495) -> ("error out"=w496:errorcluster)  [unwired: 7 in, 1 out]
        n216 = Bundle By Name(cluster=w499, "Error"=w496) -> (w498:T4)
      }
      frame "UI :F_Oper - FP Refresh" {
        # ">> Notes: 前面板刷新；<<"
        n217 = Unbundle By Name(w506) -> ("Local VIRef"=w502:refnum<vi>, "Error"=w504:errorcluster)
        n218 = call <vilib>:"PSGEN_Front Panel Delay.vi"("error in (no error)"=w504, "Delay?"=FALSE ("Defer"), "VI"=w502) -> ("error out"=w503:errorcluster)  [unwired: 7 in, 1 out]
        n219 = Bundle By Name(cluster=w506, "Error"=w503) -> (w505:T4)
      }
      frame "UI :F_Oper - Update VCH List" {
        n220 = Unbundle By Name(w515) -> ("Ref.VCHList"=w513:refnum<vi>, "Error"=w510:errorcluster)
        n221 = call "PSVCH_Core Data.vi"("Oper"=enum16{"Init", "Read", "Write"}."Read", "Error In (no error)"=w510) -> ("Error Out"=w511:errorcluster, "VCH Out"=w509:T13)  [unwired: 8 in]
        n222 = call "PSAE_VCH_Update VCH List.vi"("Error In (no error)"=w511, "VCH"=w509, "VCH Ref"=w513) -> ("Error Out"=w512:errorcluster)  [unwired: 8 in]
        n223 = Bundle By Name(cluster=w515, "Error"=w512) -> (w514:T4)
      }
      frame "UI :F_Oper - View" {
        w526 = u16 0 items=["Single"=0, "Reentrant"=8] ("Type")
        # ">> Notes: 调用显示Demo显示选择的通道数据；<<"
        n224 = Unbundle By Name(w532) -> ("Error"=w518:errorcluster)
        n225 = call "PSVCH_Core Data.vi"("Error In (no error)"=w518) -> ("Error Out"=w519:errorcluster, "VCH Out"=w517:T13)  [unwired: 9 in]
        n226 = call "PSAE_VCH_Get VCHs Enabled.vi"("Error In (no error)"=w519, "VCH"=w517) -> ("Error Out"=w529:errorcluster, "VCH"=w530:T13)  [unwired: 8 in]
        n227 = vi-ref "PSVCH_Demo_View.vi"() -> (w524:refnum<vi>)
        n228 = Unbundle By Name(w530) -> ("Tag"=w523:string[], "Time"=w521:i64[])
        n229 = Index Array(array=w521) -> (element=w520:i64)  [unwired: 1 in]
        n230 = Bundle("Tag"=w523, "Time"=w520) -> (w522:cluster{"Tag":string[], "Time":i64})  [unwired: 1 in]
        n231 = To Variant(anything=w522) -> (Variant=w525:variant)
        n232 = call "PSVCH_Load Thread.vi"("Type"=w526, "Open FP? (F)"=TRUE, "Error In"=w529, "Control Value"=w525, "VIRef"=w524) -> ("Error Out"=w528:errorcluster)  [unwired: 5 in, 1 out]
        n233 = Bundle By Name(cluster=w532, "Error"=w528) -> (w531:T4)
      }
      frame "----------VCH----------" {
        n234 = Unbundle By Name(w536) -> ("Error"=w534:errorcluster)
        n235 = Bundle By Name(cluster=w536, "Error"=w534) -> (w535:T4)
      }
      frame "UI :F_Oper - Load VCH EG" {
        n236 = Unbundle By Name(w546) -> ("Q_Local.Name"=w539:string, "Error"=w544:errorcluster)
        n237 = To Variant(anything=w539) -> (Variant=w538:variant)
        n238 = vi-ref "PSVCH_Engine.vi"() -> (w542:refnum<vi>)
        n239 = call <vilib>:"PSARC_Static Call_Single.vi"("open front panel? (F)"=FALSE ("open front panel? (T)"), "error in (no error)"=w544, "parameter else"=w538, "control name"="Q-Caller", "VI Refnum"=w542) -> ("error out"=w543:errorcluster)  [unwired: 3 in, 3 out]
        n240 = Bundle By Name(cluster=w546, "Error"=w543) -> (w545:T4)
      }
    }
    n241 = Unbundle By Name(w31) -> ("Exit"=w30:bool)
  }
  n242 = while {
    shift-right: [w553] -> w8
    shift-left: w26 -> [w550]
    tunnel: w12 -> [w549]
    tunnel: [w548] -> w9
    stop <- w552 stop-if-true
    # "Pansino Architecture - Producer Loop - Respone The UI Events"
    n243 = Unbundle By Name(w550) -> ("Error"=w551:errorcluster)
    n244 = case shown="无错误" w551 {
      tunnel: w550 -> [w557 w642]
      tunnel: [w556 w641] -> w553
      tunnel: w549 -> [w555 w638]
      tunnel: [w554 w638] -> w548
      frame No Error {
        n245 = event shown="[0] 超时" {
          selector: w555 -> [_ _ _ _ _]
          dyn-events: [_ _ _ _ _] -> w554
          timeout: 10 -> [_ _ _ _ _]
          tunnel: w557 -> [w560 w567 w583 w612 w630]
          tunnel: [w562 w566 w582 w611 w629] -> w556
          event Timeout {
            n246 = event-data() -> ()  [unwired: 1 in, 1 out]
            n247 = Unbundle By Name(w560) -> ("Q_Local.Name"=w559:string)
            n248 = call-poly <vilib>:"PSARC_Queue Management.vi"("Queue Name(unamed)"=w559) -> ("Not Exist?"=w561:bool)  [unwired: 8 in, 2 out]
            n249 = Bundle By Name(cluster=w560, "Exit"=w561) -> (w562:T4)
          }
          event Panel Close? {
            n250 = event-data() -> ()  [unwired: 1 in, 1 out]
            n251 = Unbundle By Name(w567) -> ("Q_Local.Name"=w563:string, "Error"=w568:errorcluster)
            n252 = call-poly <vilib>:"PSARC_Queue Management.vi"("error in (no error)"=w568, "Event"="UI :L_Evnt - Exit", "Queue Name(unamed)"=w563) -> ("error out"=w565:errorcluster)  [unwired: 7 in, 1 out]
            n253 = Bundle By Name(cluster=w567, "Error"=w565) -> (w566:T4)
            n254 = event-data("Discard?"=TRUE ("放弃？")) -> ()  [unwired: 1 in, 1 out]
          }
          event "View", "Run", "Pause", "Stop", "Config": Value Change {
            n255 = event-data() -> ("CtlRef"=w578:refnum<vi>)  [unwired: 1 in]
            n256 = Unbundle By Name(w583) -> ("Q_Local.Name"=w580:string, "Error"=w579:errorcluster)
            n257 = property class="Bool"(reference=w578, error in=w579) -> (reference out=w574:refnum<vi>, error out=w573:errorcluster, "Label.Text"=w575:string)
            n258 = case shown="默认" w575 {
              selector: w575 -> [w585 w594]
              tunnel: w574 -> [w587 w601]
              tunnel: w573 -> [w586 w600]
              tunnel: [w586 w589] -> w572
              tunnel: [w587 w590] -> w571
              tunnel: [w585 w593] -> w570
              frame Default {
              }
              frame "Pause*" {
                w597 = "暂停"
                n259 = property class="Bool"(reference=w601, error in=w600) -> (reference out=w591:refnum<vi>, error out=w592:errorcluster, "BoolText.Text"=w599:string)
                n260 = Equal?(x=w599, y=w597) -> (x = y?=w596:bool)
                n261 = Select(t="继续", s=w596, f=w597) -> (s? t:f=w588:string)
                n262 = Select(t=w594, s=w596, f="Continue") -> (s? t:f=w593:string)
                n263 = property class="Bool"(reference=w591, error in=w592, "BoolText.Text"=w588) -> (reference out=w590:refnum<vi>, error out=w589:errorcluster)
              }
            }
            n264 = invoke class="Bool" method="Reinit To Default"(reference=w571, error in=w572) -> (error out=w576:errorcluster)  [unwired: 1 in, 2 out]
            n265 = To Variant(anything=w570) -> (Variant=w577:variant)
            n266 = call-poly <vilib>:"PSARC_Queue Management.vi"("error in (no error)"=w576, "Data"=w577, "Event"="UI :L_Evnt - Button Click", "Queue Name(unamed)"=w580) -> ("error out"=w581:errorcluster)  [unwired: 6 in, 1 out]
            n267 = Bundle By Name(cluster=w583, "Error"=w581) -> (w582:T4)
          }
          event User Event {
            n268 = event-data() -> ("Valid?"=w608:bool, "Value Changed?"=w607:bool, "Popup Value"=w606:variant, "Call Data"=w605:variant)  [unwired: 1 in]
            n269 = Unbundle By Name(w612) -> ("Q_Local.Name"=w609:string, "Error"=w602:errorcluster)
            n270 = And(x=w608, y=w607) -> (x .and. y?=w604:bool)
            n271 = Bundle("Popup Value"=w606, "Call Data"=w605) -> (w603:T6)  [unwired: 1 in]
            n272 = case shown="真" w604 {
              tunnel: [w613 w618] -> w610
              tunnel: w609 -> [_ w617]
              tunnel: w602 -> [w613 w616]
              tunnel: w603 -> [_ w614]
              frame False {
              }
              frame True {
                n273 = To Variant(anything=w614) -> (Variant=w615:variant)
                n274 = call-poly <vilib>:"PSARC_Queue Management.vi"("error in (no error)"=w616, "Data"=w615, "Event"="UI :L_Evnt - Popup Event", "Queue Name(unamed)"=w617) -> ("error out"=w618:errorcluster)  [unwired: 6 in, 1 out]
              }
            }
            n275 = Bundle By Name(cluster=w612, "Error"=w610) -> (w611:T4)
          }
          event "VCH": Mouse Down? {
            n276 = event-data() -> ("CtlRef"=w623:refnum<vi>, "Coords"=w625:T16)  [unwired: 1 in]
            n277 = Unbundle By Name(w630) -> ("PopUp Name"=w624:string, "Q_Local.Name"=w627:string, "Error"=w626:errorcluster)
            n278 = property class="Tree (严格)"(reference=w623) -> ("DisabledEnum"=w622:T5)  [unwired: 1 in, 2 out]
            n279 = Equal?(x=T5."Enabled", y=w622) -> (x = y?=w620:bool)
            n280 = case shown="真" w620 {
              tunnel: [w631 w637] -> w628
              tunnel: w627 -> [_ w636]
              tunnel: w626 -> [w631 w635]
              tunnel: w625 -> [_ w634]
              tunnel: w624 -> [_ w633]
              tunnel: w623 -> [_ w632]
              frame False {
              }
              frame True {
                n281 = call "PSAE_VCH_Popup Judge.vi"("PopUp Name"=w633, "Error In (no error)"=w635, "Name"=w636, "Coords"=w634, "TreeRef"=w632) -> ("Error Out"=w637:errorcluster)  [unwired: 6 in]
              }
            }
            n282 = Bundle By Name(cluster=w630, "Error"=w628) -> (w629:T4)
            n283 = event-data() -> ()  [unwired: 2 in, 1 out]
          }
        }
      }
      frame Error {
        n284 = Unbundle By Name(w642) -> ("Q_Local.Name"=w640:string, "Error"=w639:errorcluster)
        n285 = call-poly <vilib>:"PSARC_Queue Management.vi"("Queue Name(unamed)"=w640) -> ("Not Exist?"=w643:bool)  [unwired: 8 in, 2 out]
        n286 = case shown="假" w643 {
          selector: w643 -> [_ w651]
          tunnel: w642 -> [w649 w653]
          tunnel: [w645 w652] -> w641
          tunnel: w639 -> [w646 _]
          tunnel: w640 -> [w648 _]
          frame False {
            n287 = To Variant(anything=w646) -> (Variant=w647:variant)
            n288 = call-poly <vilib>:"PSARC_Queue Management.vi"("Data"=w647, "Event"="THx :C_Resp - Error", "Queue Name(unamed)"=w648) -> ("error out"=w644:errorcluster)  [unwired: 7 in, 1 out]
            n289 = Bundle By Name(cluster=w649, "Error"=w644) -> (w645:T4)
          }
          frame True {
            n290 = Bundle By Name(cluster=w653, "Exit"=w651) -> (w652:T4)
          }
        }
      }
    }
    n291 = Unbundle By Name(w553) -> ("Exit"=w552:bool)
  }
  n292 = Unbundle By Name(w8) -> ("PopUp Name"=w3:string, "Error"=w11:errorcluster)
  n293 = Unbundle By Name(w21) -> ("Q_Local.Name"=w24:string, "Error"=w22:errorcluster)
  n294 = disable-structure shown="禁用" {
    frame Disabled {
    }
    frame Enabled {
    }
  }
  n295 = call-poly <vilib>:"PSARC_Queue Management.vi"("error in (no error)"=w22, "Queue Name(unamed)"=w24) -> ()  [unwired: 7 in, 3 out]
  n296 = Unregister For Events(event registration refnum=w9, error in=w11) -> (error out=w10:errorcluster)
  n297 = call <vilib>:"PSPOP_Close.vi"("Name"=w3, "error in (no error)"=w10) -> ("error out"=w7:errorcluster)  [unwired: 9 in]
  n298 = call <vilib>:"Clear Errors.vi"("error in (no error)"=w7) -> ()  [unwired: 5 in, 2 out]
